vi "Debug_Convert_Data_to_String.vi"(8 "error in (no error)":errorcluster, 11 "AB_Build in":refnum<class "AB_Build.lvclass">) -> (0 "error out":errorcluster, 2 "classData":string, 3 "AB_Build out":refnum<class "AB_Build.lvclass">)   [LabVIEW 2020, in "AB_Build.lvclass"]
uses:
  <vilib>/AppBuilder/AB_Classes/Build/AB_Build.lvclass
  <vilib>/AppBuilder/AB_Classes/Build/AB_Build.lvclass/AB_Build.ctl
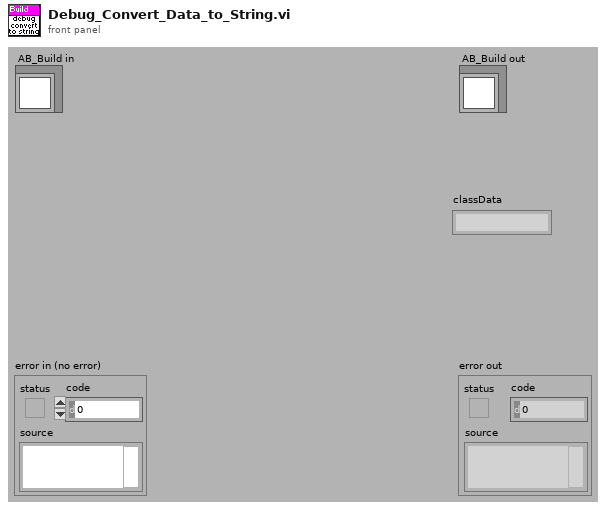
[diagram p1: front panel]
types:
  T1 = typedef "ItemRef.ctl" = u64
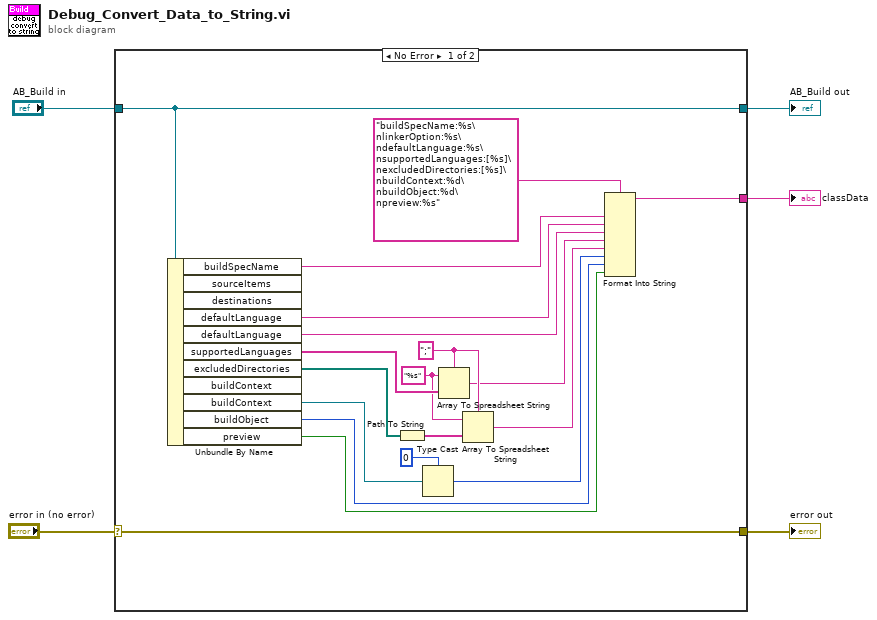
[diagram p0: block diagram]
diagram:
  n1 = case shown="No Error" "error in (no error)" {
    selector: "error in (no error)" -> [w24 w26]
    tunnel: [w24 w26] -> w4
    tunnel: [w23 w25] -> w2
    tunnel: "AB_Build in" -> [w23 w25]
    tunnel: [w6 _] -> w1
    frame No Error {
      w14 = ";" ("delimiter (Tab)")
      w15 = "%s" ("format string")
      n2 = Unbundle By Name(w23) -> ("buildSpecName"=w21:string, "defaultLanguage"=w20:string, "defaultLanguage"=w19:string, "supportedLanguages"=w18:string[], "excludedDirectories"=w17:path[], "buildContext"=w11:refnum<vi>, "buildObject"=w8:T1, "preview"=w7:bool)  [unwired: 3 out]
      n3 = Path To String(path=w17) -> (string=w16:string[])
      n4 = Type Cast(type=u64 0, x=w11) -> (*(type *) &x=w9:u64)
      n5 = Array To Spreadsheet String(delimiter (Tab)=w14, array=w18, 3:w15) -> (spreadsheet string=w12:string)
      n6 = Array To Spreadsheet String(delimiter (Tab)=w14, array=w16, 3:w15) -> (spreadsheet string=w13:string)
      n7 = Format Into String(format string="buildSpecName:%s\nlinkerOption:%s\ndefaultLanguage:%s\nsupportedLanguages:[%s]\nexcludedDirectories:[%s]\nbuildContext:%d\nbuildObject:%d\npreview:%s", w21, w20, w19, w12, w13, w9, w8, w7) -> (resulting string=w6:string)  [unwired: 2 in, 1 out]
    }
    frame Error {
    }
  }
  "error out" <- w4
  "AB_Build out" <- w2
  "classData" <- w1
